vi "Set RHS.vi"(7 "target RHS":refnum<class "NI_RHS.lvclass">, 8 "error in (no error)":errorcluster, 10 "RHS":variant, 11 "PDE in":refnum<class "NI_PDE.lvclass">) -> (0 "error out":errorcluster, 3 "PDE out":refnum<class "NI_PDE.lvclass">)   [LabVIEW 2017, in "NI_PDE.lvlib" / "NI_PDE.lvclass"]
uses:
  <vilib>/gmath/pde.llb/PDEClass/NI_PDE.lvclass
  <vilib>/gmath/pde.llb/RHSClass/NI_RHS.lvclass
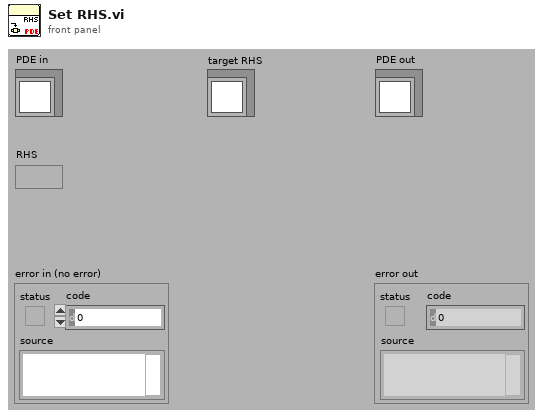
[diagram p1: front panel]
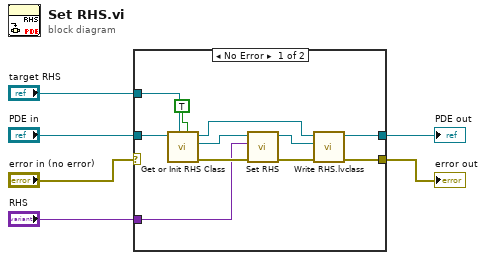
[diagram p0: block diagram]
diagram:
  n1 = case shown="No Error" "error in (no error)" {
    selector: "error in (no error)" -> [_ w19]
    tunnel: "PDE in" -> [w17 w18]
    tunnel: [w15 w18] -> w6
    tunnel: [w14 w19] -> w5
    tunnel: "target RHS" -> [w13 _]
    tunnel: "RHS" -> [w8 _]
    frame No Error {
      n2 = call <vilib>:"Get or Init RHS Class.vi"("type check? (T)"=TRUE, "target RHS"=w13, "PDE out"=w17) -> ("error out"=w12:errorcluster, "RHS out"=w11:refnum<class "NI_RHS.lvclass">, "PDE in"=w16:refnum<class "NI_PDE.lvclass">)  [unwired: 1 in, 5 out]
      n3 = call-dynamic "Set RHS.vi"("error in (no error)"=w12, "RHS"=w8, "RHS in"=w11) -> ("error out"=w9:errorcluster, "RHS out"=w10:refnum<class "NI_RHS.lvclass">)  [unwired: 7 out]
      n4 = call-dynamic "Write RHS.lvclass.vi"("error in (no error)"=w9, "RHS.lvclass"=w10, "PDE.lvclass in"=w16) -> ("error out"=w14:errorcluster, "PDE.lvclass out"=w15:refnum<class "NI_PDE.lvclass">)  [unwired: 7 out]
    }
    frame Error {
    }
  }
  "PDE out" <- w6
  "error out" <- w5
